vi "PH_gentec_P-Link.PC Write PSDB.vi"(0 "i ref in":refnum<vi>, 5 "error IO":errorcluster) -> (14 "i ref out":refnum<vi>, 19 "error out":errorcluster)   [LabVIEW 2014, in "PH_gentec_P-Link.lvlib"]
doc: "This is the proc case which writes data to the PHELIX shot data base."
uses:
  PH_gentec_P-Link.lvlib
  PH_Basics/PH_PSDBWriter/PH_PSDBWriter.lvlib
  PH_Basics/PH_Powermeter_BaseClass/PH_Powermeter_BaseClass.lvlib
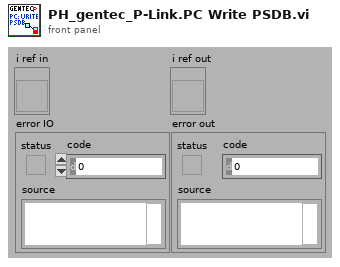
[diagram p1: front panel]
types:
  T1 = typedef "PH_Powermeter_BaseClass.lvlib/PH_Powermeter_BaseClass.i attribute.ctl" = cluster{"GUI References":T2, "Connection":T3, "Head Attributes":T5, "VISA resource":refnum<visa-resource-name>, "Energy":T6, "Service ID Energy":i32, "Wanted Settings":T7, "Current Settings":T7}
  T2 = typedef "PH_Powermeter_BaseClass.lvlib/PH_Powermeter_BaseClass.GUI Refs.ctl" = cluster{"Head Attributes":refnum<vi>, "Energy":refnum<vi>, "Connection":refnum<vi>, "VISA Resource":refnum<vi>, "Scaling Factor":refnum<vi>, "Range":refnum<vi>, "Wavelength":refnum<vi>, "Trigger Level":refnum<vi>, "Wanted Settings":refnum<vi>, "Current Settings":refnum<vi>}
  T3 = typedef "PH_Powermeter_BaseClass.lvlib/PH_Powermeter_BaseClass.Connection.ctl" = cluster{"failed checks":i8, "Timeout":bool, "Data read":string, "Failure":bool, "Error":bool, "State":T4}
  T4 = typedef "PH_Powermeter_BaseClass.lvlib/PH_Powermeter_BaseClass.State.ctl" = enum32{"off", "operating", "opened", "checked", "connected", "Sets to change", "running"}
  T5 = typedef "PH_Powermeter_BaseClass.lvlib/PH_Powermeter_BaseClass.Head Attributes.ctl" = cluster{"Instrument Type":string, "Head Version":string, "Head Name":string, "Serial Number":string, "Firmware":string, "Sensor Type":string, "MinimumRange":u32, "Maximum Range":u32, "Min Wavelength":i32, "Max Wavelength":i32}
  T6 = typedef "PH_Powermeter_BaseClass.lvlib/PH_Powermeter_BaseClass.Energy.ctl" = cluster{"current Value":dbl, "unscaled":dbl, "Scaling Factor":dbl}
  T7 = typedef "PH_Powermeter_BaseClass.lvlib/PH_gentec_BaseClass.Head Settings.ctl" = cluster{"Trigger Level":dbl, "Wavelength":u32, "Range":u32}
  T8 = typedef "PH_PSDBWriter.lvlib/PH_PSDBWriter.Numeric dataset.ctl" = cluster{"name":string, "data":dbl, "unit":string}
  T9 = typedef "PH_PSDBWriter.lvlib/PH_PSDBWriter.String dataset.ctl" = cluster{"name":string, "data":string, "unit":string}
  T10 = typedef "PH_PSDBWriter.lvlib/PH_PSDBWriter.PSDB Dataset.ctl" = cluster{"Version":i32, "2D data Input":T11[], "Boolean Input":T13[], "Image Input":T14[], "Numeric Input":T8[], "String Input":T9[]}
  T11 = typedef "PH_PSDBWriter.lvlib/PH_PSDBWriter.2D dataset.ctl" = cluster{"name":string, "data":dbl[][], "axis description":T12}
  T12 = typedef "PSDB.lvlib/PSDB_AxisDescription.ctl" = cluster{"x axis label":string, "y axis label":string, "x axis unit":string, "y axis unit":string}
  T13 = typedef "PH_PSDBWriter.lvlib/PH_PSDBWriter.Boolean dataset.ctl" = cluster{"name":string, "data":bool, "unit":string}
  T14 = typedef "PH_PSDBWriter.lvlib/PH_PSDBWriter.Image dataset.ctl" = cluster{"name":string, "data":T15, "unit":string}
  T15 = typedef "IMAQ Image.ctl" = refnum<image>
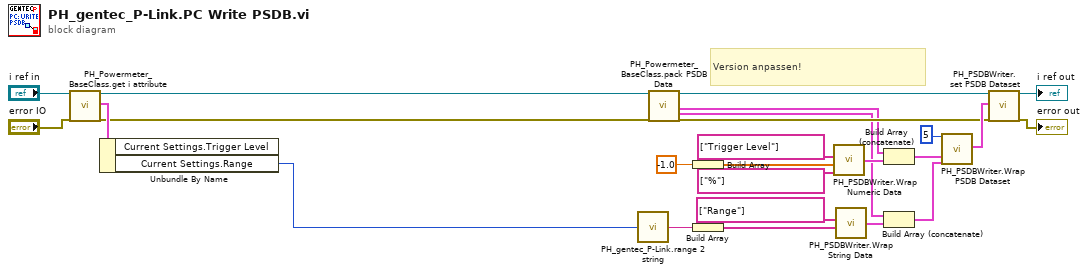
[diagram p0: block diagram]
diagram:
  # "Version anpassen!"
  n1 = call "PH_Powermeter_BaseClass.get i attribute.vi"("i ref in"="i ref in", "error in (no error)"="error IO") -> ("i ref out"=w3:refnum<vi>, "i attribute"=w5:T1, "error out"=w2:errorcluster)  [unwired: 15 in]
  n2 = Unbundle By Name(w5) -> ("Current Settings.Range"=w4:u32)  [unwired: 1 out]
  n3 = call "PH_gentec_P-Link.range 2 string.vi"("Range"=w4) -> ("Range as string"=w7:string)
  n4 = call "PH_Powermeter_BaseClass.pack PSDB Data.vi"("i ref in"=w3, "error IO"=w2) -> ("i ref out"=w13:refnum<vi>, "PSDB Numeric Data Array"=w9:T8[], "PSDB String Data Array"=w8:T9[], "error out"=w12:errorcluster)  [unwired: 14 in]
  n5 = Build Array(-1.0 ("f")) -> (w15:dbl[])
  n6 = Build Array(w7) -> (w17:string[])
  n7 = call "PH_PSDBWriter.Wrap Numeric Data.vi"("Unit Array"=string[] ["%"], "Data Array"=w15, "Name Array"=string[] ["Trigger Level"]) -> ("PSDB Numeric Data Array"=w22:T8[])  [unwired: 1 in]
  n8 = call "PH_PSDBWriter.Wrap String Data.vi"("Data Array"=w17, "Name Array"=string[] ["Range"]) -> ("PSDB String Data Array"=w21:T9[])  [unwired: 2 in]
  n9 = Build Array (concatenate)(w9, w22) -> (w11:T8[])
  n10 = Build Array (concatenate)(w8, w21) -> (w10:T9[])
  n11 = call "PH_PSDBWriter.Wrap PSDB Dataset.vi"("Version"=5, "Numeric Input"=w11, "String Input"=w10) -> ("PSDB Dataset"=w19:T10)  [unwired: 16 in]
  n12 = call "PH_PSDBWriter.set PSDB Dataset.vi"("VI in"=w13, "PSDB Dataset"=w19, "error in (no error)"=w12) -> ("VI out"=→"i ref out":refnum<vi>, "error out"=→"error out":errorcluster)  [unwired: 15 in]
